vi "RandomUnitVector.vi"(10 "Old 3D Unit Vector":cluster{"X":dbl, "Y":dbl, "Z":dbl}, 11 "G":dbl=nan) -> (2 "Random 3D Unit Vector":cluster{"X":dbl, "Y":dbl, "Z":dbl}, 3 "Random 2D Unit Vector":cluster{"X":dbl, "Y":dbl})   [LabVIEW 2019]
uses:
  Random Number Within Range - DBL__ogtk.vi
panel:
  out "Waveform Chart":cluster{"[0]":dbl, "[1]":dbl, "[2]":dbl}(graph)
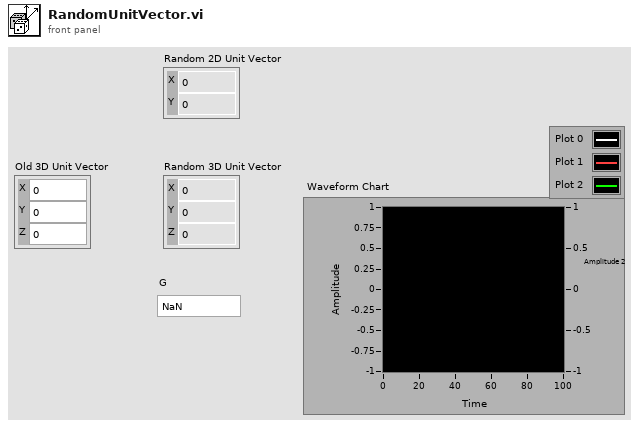
[diagram p1: front panel]
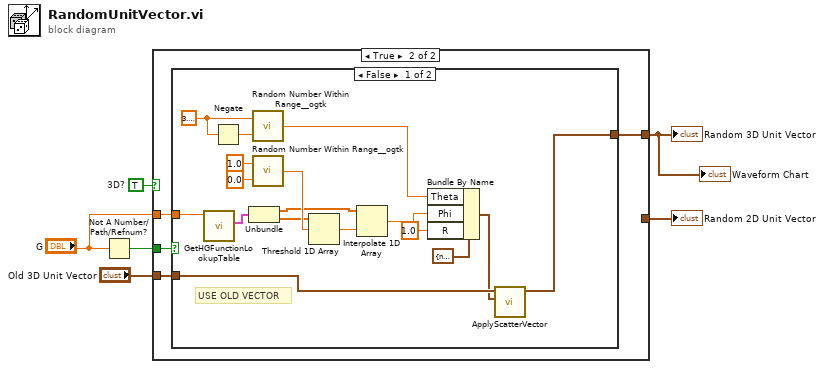
[diagram p0: block diagram]
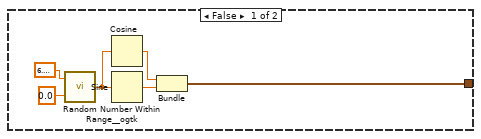
[diagram p2: hidden frame]
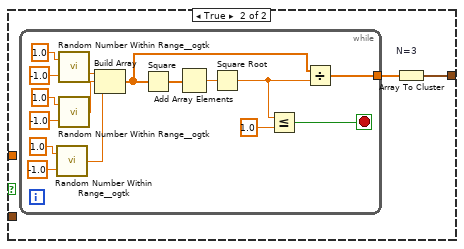
[diagram p3: hidden frame]
diagram:
  w5 = TRUE  # 3D?
  n1 = Not A Number/Path/Refnum?(number/path/refnum="G") -> (NaN/Path/Refnum?=w4:bool)
  n2 = case shown="True" w5 {
    tunnel: [_ w16] -> w2
    tunnel: [w7 _] -> w6
    tunnel: w4 -> [_ w15]
    tunnel: "G" -> [_ w14]
    tunnel: "Old 3D Unit Vector" -> [_ w13]
    frame False {
      n3 = call-poly "Random Number Within Range__ogtk.vi"("High"=6.283185307179586, "Low"=0.0) -> ("Random Number"=w10:dbl)  [unwired: 3 in]
      n4 = Cosine(x=w10) -> (cos(x)=w9:dbl)
      n5 = Sine(x=w10) -> (sin(x)=w8:dbl)
      n6 = Bundle(w9, w8) -> (w7:cluster{dbl, dbl})  [unwired: 1 in]
    }
    frame True {
      n7 = case shown="False" w15 {
        tunnel: [w17 w34] -> w16
        tunnel: w14 -> [w33 _]
        tunnel: w13 -> [w19 _]
        frame False {
          w26 = 3.141592653589793
          # "USE OLD VECTOR"
          n8 = call "GetHGFunctionLookupTable.vi"("G"=w33) -> ("Integrated Distribution"=w21:cluster{dbl[], dbl[]})  [unwired: 9 in, 1 out]
          n9 = Negate(x=w26) -> (-x=w25:dbl)
          n10 = Unbundle(w21) -> (w22:dbl[], w23:dbl[])
          n11 = call-poly "Random Number Within Range__ogtk.vi"("High"=w26, "Low"=w25) -> ("Random Number"=w24:dbl)  [unwired: 3 in]
          n12 = call-poly "Random Number Within Range__ogtk.vi"("High"=1.0, "Low"=0.0) -> ("Random Number"=w31:dbl)  [unwired: 3 in]
          n13 = Threshold 1D Array(2:w31, 3:w23) -> (0:w30:dbl)  [unwired: 1 in]
          n14 = Interpolate 1D Array(1:w30, 2:w22) -> (0:w28:dbl)
          n15 = Bundle By Name(cluster=cluster{"R":dbl, "Theta":dbl, "Phi":dbl} {"R"=nan, "Theta"=nan, "Phi"=nan} ("Spherical Coordinates In"), "Theta"=w24, "Phi"=w28, "R"=1.0) -> (w18:cluster{"R":dbl, "Theta":dbl, "Phi":dbl})
          n16 = call "ApplyScatterVector.vi"("Scatter Coordinates (Spherical)"=w18, "Old Velocity Vector (X,Y,Z)"=w19) -> ("New Velocity Vector (X,Y,Z)"=w17:cluster{"X":dbl, "Y":dbl, "Z":dbl})  [unwired: 9 in]
        }
        frame True {
          n17 = while {
            tunnel: [w45] -> w35
            stop <- w48 stop-if-true
            n18 = call-poly "Random Number Within Range__ogtk.vi"("High"=1.0 ("Low"), "Low"=-1.0) -> ("Random Number"=w36:dbl)  [unwired: 3 in]
            n19 = call-poly "Random Number Within Range__ogtk.vi"("High"=1.0 ("Low"), "Low"=-1.0) -> ("Random Number"=w38:dbl)  [unwired: 3 in]
            n20 = call-poly "Random Number Within Range__ogtk.vi"("High"=1.0 ("Low"), "Low"=-1.0) -> ("Random Number"=w37:dbl)  [unwired: 3 in]
            n21 = Build Array(w38, w37, w36) -> (w46:dbl[])
            n22 = Square(x=w46) -> (x^2=w50:dbl[])
            n23 = Add Array Elements(numeric array=w50) -> (sum=w51:dbl)
            n24 = Square Root(x=w51) -> (sqrt(x)=w47:dbl)
            n25 = Less Or Equal?(x=w47, y=1.0) -> (x <= y?=w48:bool)
            n26 = Divide(x=w46, y=w47) -> (x/y=w45:dbl[])
          }
          n27 = Array To Cluster "N=3"(array=w35) -> (cluster=w34:cluster{"[0]":dbl, "[1]":dbl, "[2]":dbl})
        }
      }
    }
  }
  "Random 3D Unit Vector" <- w2
  "Random 2D Unit Vector" <- w6
  "Waveform Chart" <- w2
